vi "Save QOI Image (UTF-8 Path).vi"(8 "error in (no error)":errorcluster, 10 "Image":T1, 11 "Path In":string) -> (0 "error out":errorcluster, 3 "Path Out":string)   [LabVIEW 2020, in "G-Image.lvlib"]
doc: "Saves an image in QOI format to disk."
uses:
  G-Image.lvlib
  <vilib>/picture/picture.llb/imagedata.ctl
  Controls/Image Save Format.ctl
  84b65850-7e2c-4555-ae76-2c591eca4b86.vi
  Private/Result To Error.vi
  Private/Get Image Data.vi
  Private/ARGB To RGBA.vi
  Private/Depth To Number Channels.vi
  Image Processing/To True Color Image.vi
  <vilib>/Utility/error.llb/Error Cluster From Error Code.vi
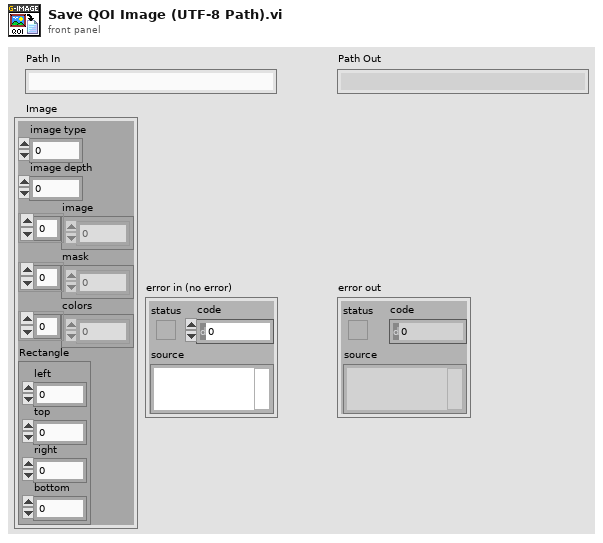
[diagram p1: front panel]
types:
  T1 = typedef "imagedata.ctl" = cluster{"image type":i32, "image depth":i32, "image":u8[], "mask":u8[], "colors":u32[], "Rectangle":cluster{"left":i16, "top":i16, "right":i16, "bottom":i16}}
  T2 = typedef "G-Image.lvlib/Image Save Format.ctl" = enum16{"png", "jpg", "bmp", "gif", "tga", "qoi"}
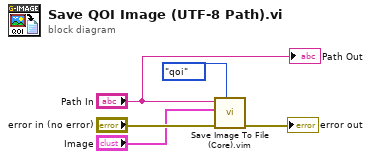
[diagram p0: block diagram]
diagram:
  n1 = call "Save Image To File (Core).vim"("Save Format"=Image_Save_Format."qoi", "error in (no error)"="error in (no error)", "Picture"="Image", "Path In"="Path In") -> ("error out"=→"error out":errorcluster)  [unwired: 6 in, 1 out]
  "Path Out" <- "Path In"
